vi "CallTrendPlot.vi"(8 "错误输入（无错误）":errorcluster, 10 "Y通道":string, 11 "X通道":string) -> (0 "错误输出":errorcluster, 3 "VI输出":refnum<vi>)   [LabVIEW 2018, in "DataDisplay.lvlib"]
uses:
  DataDisplay.lvlib
  UI/TrendPlot.vi
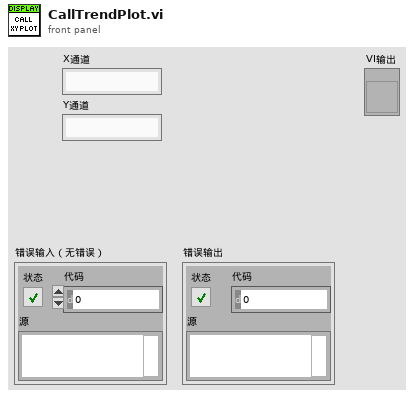
[diagram p1: front panel]
types:
  T1 = enum32{"Invalid", "Standard", "Closed", "Hidden", "Minimized", "Maximized"}
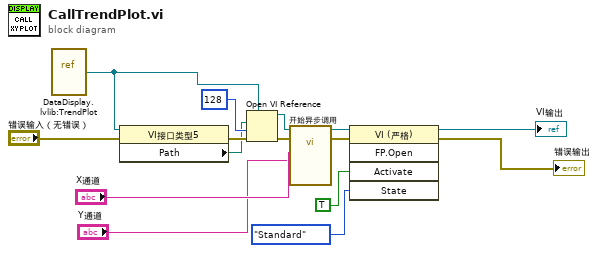
[diagram p0: block diagram]
diagram:
  n1 = vi-ref "DataDisplay.lvlib:TrendPlot.vi"() -> (w6:refnum<vi>)
  n2 = property class="VI接口类型5"(reference=w6, error in="错误输入（无错误）") -> (error out=w9:errorcluster, "Path"=w5:path)  [unwired: 1 out]
  n3 = Open VI Reference(type specifier VI Refnum (for type only)=w6, vi path=w5, options=128 ("选项"), error in (no error)=w9) -> (vi reference=w7:refnum<vi>, error out=w10:errorcluster)  [unwired: 2 in]
  n4 = call-by-ref "开始异步调用"(reference=w7, error in=w10, "Y通道"="Y通道", "X通道"="X通道") -> (reference out=w8:refnum<vi>, error out=w11:errorcluster)  [unwired: 10 in]
  n5 = invoke class="VI (严格)" method="FP.Open"(reference=w8, error in=w11, "Activate"=TRUE ("激活？"), "State"=T1."Standard" ("状态")) -> (reference out=→"VI输出":refnum<vi>, error out=→"错误输出":errorcluster)  [unwired: 1 in, 3 out]
